vi "task1000.vi"() -> ()   [LabVIEW 2020]
uses:
  <vilib>/DAQmx/read.llb/DAQmx Read (Analog 1D Wfm NChan NSamp).vi
  <vilib>/DAQmx/create/channels.llb/DAQmx Create Channel (AI-Current-Basic).vi
  <vilib>/DAQmx/configure/timing.llb/DAQmx Timing (Sample Clock).vi
  <vilib>/DAQmx/miscellaneous.llb/DAQmx Fill In Error Info.vi
panel:
  in  "index":i32
  in  "physical channels":tag
  out "Waveform Graph":waveform(dbl)[](graph)
  in  "Sampling rate":dbl
  in  "Number of sample":dbl
  in  "Min":dbl
  in  "Max":dbl
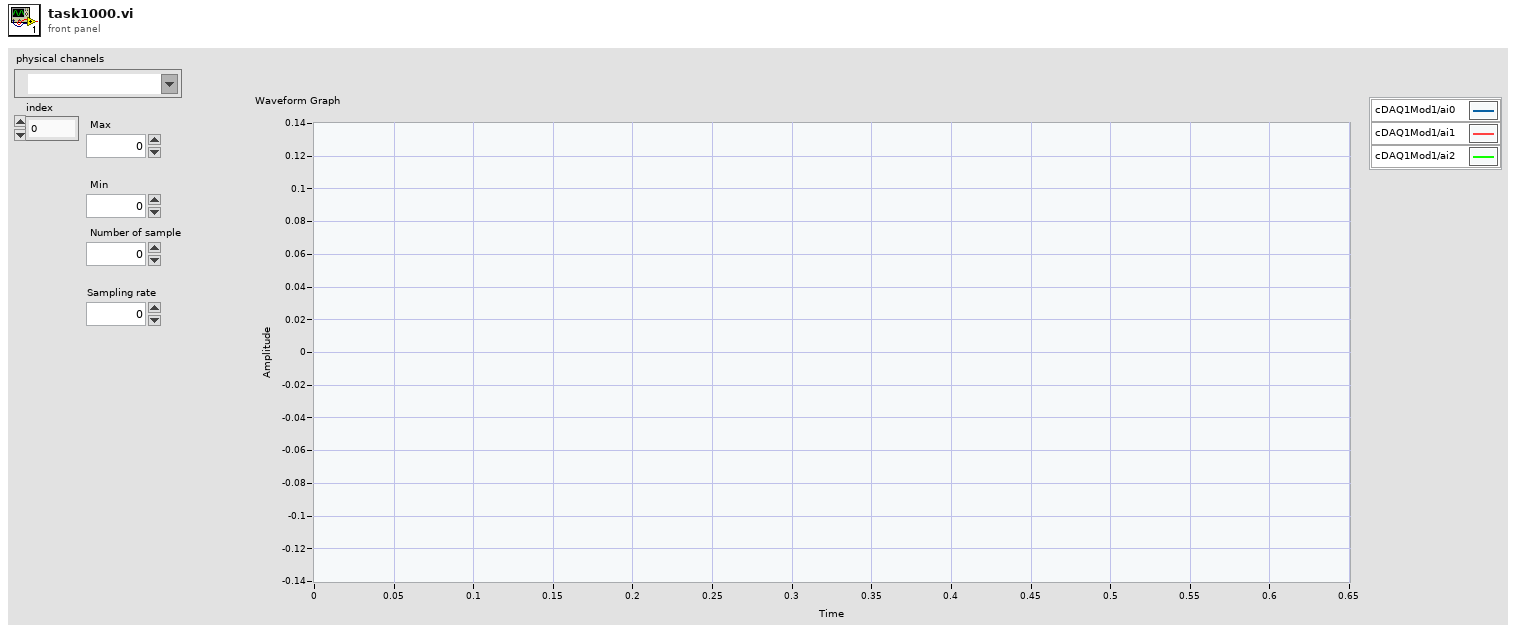
[diagram p1: front panel]
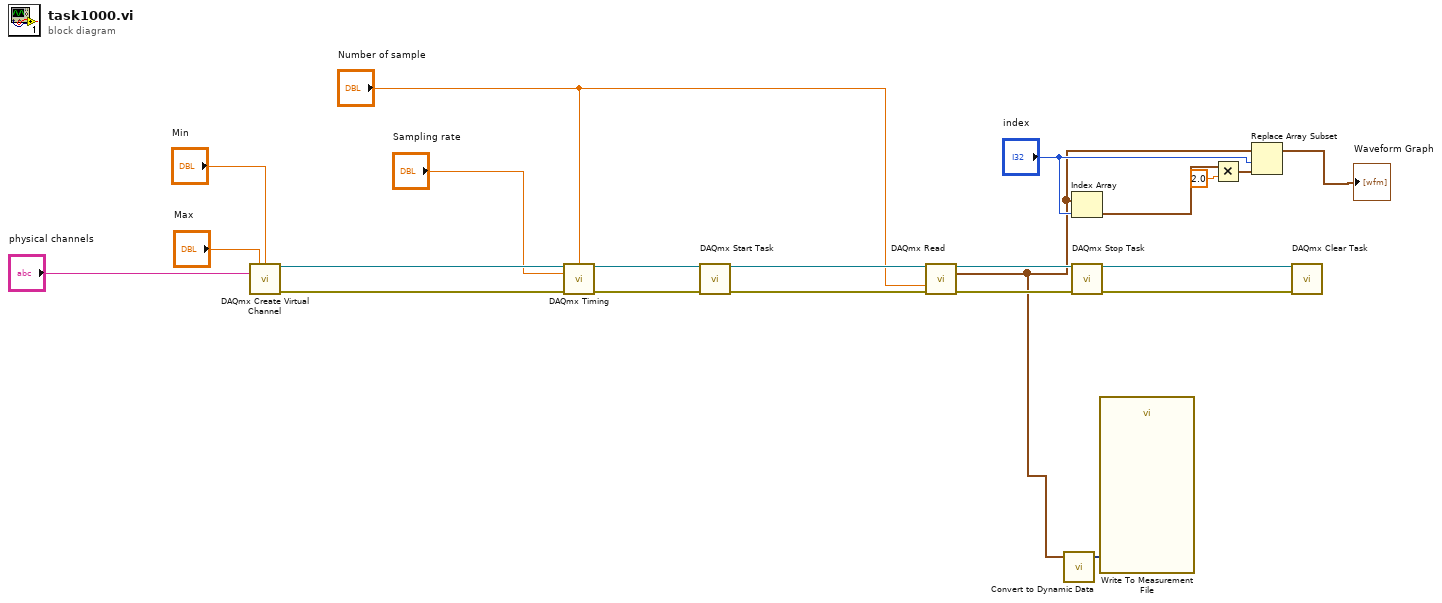
[diagram p0: block diagram]
diagram:
  n1 = call-poly <vilib>:"DAQmx Create Virtual Channel.vi"("maximum value"="Max", "minimum value"="Min", "physical channels"="physical channels") -> ("task out"=w22:refnum<k21>, "error out"=w12:errorcluster)  [unwired: 11 in]
  n2 = call-poly <vilib>:"DAQmx Timing.vi"("task/channels in"=w22, "samples per channel"="Number of sample", "rate"="Sampling rate", "error in"=w12) -> ("task out"=w21:refnum<k21>, "error out"=w11:errorcluster)  [unwired: 10 in]
  n3 = call <vilib>:"DAQmx Start Task.vi"("task/channels in"=w21, "error in"=w11) -> ("task out"=w20:refnum<k21>, "error out"=w10:errorcluster)  [unwired: 12 in]
  n4 = call-poly <vilib>:"DAQmx Read.vi"("task/channels in"=w20, "timeout"="Number of sample", "error in"=w10) -> ("task out"=w19:refnum<k21>, "data"=w1:waveform(dbl)[], "error out"=w9:errorcluster)  [unwired: 10 in]
  n5 = call "Convert to Dynamic Data"("Array"=w1) -> ("Dynamic Data Type"=w2:dynamicdata)  [unwired: 3 in]
  n6 = Index Array "Index Array"(array=w1, index="index") -> (element=w6:waveform(dbl))
  n7 = call <vilib>:"DAQmx Stop Task.vi"("task/channels in"=w19, "error in"=w9) -> ("task out"=w18:refnum<k21>, "error out"=w8:errorcluster)  [unwired: 12 in]
  n8 = call "Write To Measurement File"("Signals"=w2) -> ()  [unwired: 16 in, 3 out]
  n9 = Multiply(x=w6, y=2.0) -> (x*y=w5:waveform(dbl))
  n10 = Replace Array Subset "Replace Array Subset"(array=w1, new element=w5, index="index") -> (→"Waveform Graph":waveform(dbl)[])
  n11 = call <vilib>:"DAQmx Clear Task.vi"("task in"=w18, "error in"=w8) -> ()  [unwired: 13 in, 1 out]
